vi "Terminal_Alarm_Condition.vi"() -> (3 "试验轴承单元":T1)   [LabVIEW 2014]
uses:
  Terminal_Global_Alarm_condition.vi
  Terminal-Global-SetValues.vi
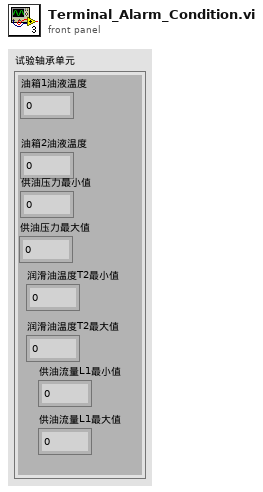
[diagram p1: front panel]
types:
  T1 = cluster{"油箱1油液温度":dbl, "油箱2油液温度":dbl, "供油压力最小值":dbl, "供油压力最大值":dbl, "润滑油温度T2最小值":dbl, "润滑油温度T2最大值":dbl, "供油流量L1最小值":dbl, "供油流量L1最大值":dbl}
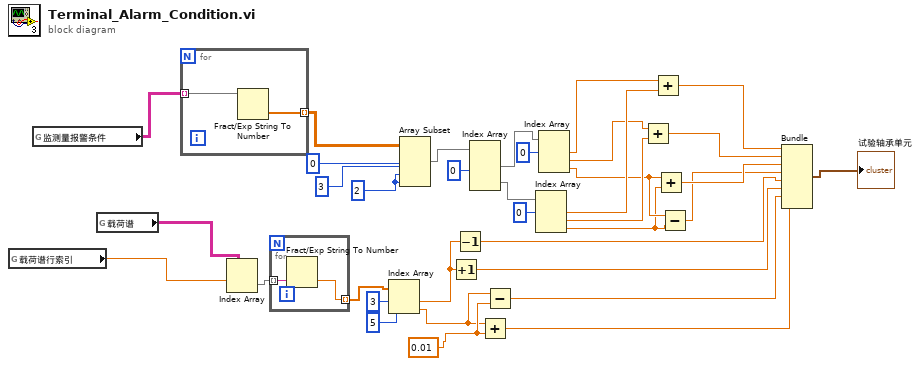
[diagram p0: block diagram]
diagram:
  w7 = 0.01
  w33 = 2 ("索引")
  n1 = global read "Terminal-Global-SetValues.vi" "载荷谱行索引"() -> (w13:dbl)
  n2 = global read "Terminal_Global_Alarm_condition.vi" "监测量报警条件"() -> (w26:string[][])
  n3 = global read "Terminal-Global-SetValues.vi" "载荷谱"() -> (w14:string[][])
  n4 = for {
    tunnel: w26 -> [w37] mode=indexing
    tunnel: [w36] -> w25 mode=indexing
    n5 = Fract/Exp String To Number(string=w37) -> (number=w36:dbl[])  [unwired: 3 in, 1 out]
  }
  n6 = Index Array(array=w14, index (row)=w13) -> (element=w10:string[])  [unwired: 1 in]
  n7 = for {
    tunnel: w10 -> [w39] mode=indexing
    tunnel: [w38] -> w9 mode=indexing
    n8 = Fract/Exp String To Number(string=w39) -> (number=w38:dbl)  [unwired: 3 in, 1 out]
  }
  n9 = Index Array(array=w9, index #1=3 ("索引"), index #2=5 ("索引")) -> (element #1=w8:dbl, element #2=w6:dbl)
  n10 = Array Subset(array=w25, index (row)=0 ("索引"), length (row)=3 ("长度"), index (col)=w33, length (col)=w33) -> (w32:dbl[][])
  n11 = Increment(x=w8) -> (x+1=w5:dbl)
  n12 = Decrement(x=w8) -> (x-1=w4:dbl)
  n13 = Index Array(array=w32, index (col) #1=0 ("禁用的索引 (列)")) -> (element #1=w30:dbl[], element #2=w29:dbl[])  [unwired: 3 in]
  n14 = Add(x=w6, y=w7) -> (x+y=w2:dbl)
  n15 = Subtract(x=w6, y=w7) -> (x-y=w3:dbl)
  n16 = Index Array(array=w29, index #1=0 ("索引")) -> (element #1=w23:dbl, element #2=w21:dbl, element #3=w19:dbl)  [unwired: 2 in]
  n17 = Index Array(array=w30, index #1=0 ("索引")) -> (element #1=w24:dbl, element #2=w22:dbl, element #3=w20:dbl)  [unwired: 2 in]
  n18 = Add(x=w22, y=w21) -> (x+y=w17:dbl)
  n19 = Add(x=w24, y=w23) -> (x+y=w18:dbl)
  n20 = Add(x=w20, y=w19) -> (x+y=w16:dbl)
  n21 = Subtract(x=w20, y=w19) -> (x-y=w15:dbl)
  n22 = Bundle(w18, w17, w16, w15, w4, w5, w3, w2) -> (→"试验轴承单元":cluster{dbl, dbl, dbl, dbl, dbl, dbl, dbl, dbl})  [unwired: 1 in]
